vi "LSMcontroller_v60_PIzstage.vi"() -> ()   [LabVIEW 2015] (continued)
                                n921 = local write "img_CH2"(w3215) -> ()
                                n922 = local write "photons/frame"(w3208) -> ()
                                n923 = Array Max & Min(array=w3210) -> (max value=w3211:u16)  [unwired: 3 out]
                                n924 = To Single Precision Float(number=w3210) -> (single precision float=w3213:sgl[][])
                                n925 = case shown="True" w3222 {
                                tunnel: w3221 -> [_ w3226]
                                frame False {
                                }
                                frame True {
                                n926 = Quotient & Remainder(x=w3226, y=u32 2 ("min phot")) -> (floor(x/y)=w3225:u32)  [unwired: 1 out]
                                n927 = Max & Min(x=w3225, y=u32 5) -> (max(x,y)=w3224:u32)  [unwired: 1 out]
                                n928 = local write "min phot"(w3224) -> ()
                                }
                                }
                                n929 = To Double Precision Float(number=w3211) -> (double precision float=w3212:dbl)
                                n930 = local write "img_CH1"(w3213) -> ()
                                n931 = property on="img_CH1" class="IntGraph (strict)"("ZScale.Maximum"=w3212) -> ()  [unwired: 2 in, 2 out]
                                }
                                }
                                }
                                frame #4 {
                                w3230 = u16 1 items=["Stream to disk", "Post process", "real time process"] ("Ring")
                                n932 = local read "T3R Data processing"() -> (w3229:u16)
                                n933 = Equal?(x=w3229, y=w3230) -> (x = y?=w3228:bool)
                                n934 = case shown="False" w3228 {
                                frame False {
                                # "intensity"
                                n935 = local read "Current Average"() -> (w3235:sgl)
                                n936 = local read "image2list"() -> (w3231:u16)
                                n937 = local read "image1list"() -> (w3232:u16)
                                n938 = call "dattoimage.vi"("image2list"=w3231, "Current Average"=w3235, "image1list"=w3232) -> ("image 1 array out"=w3234:sgl[][])  [unwired: 1 out]
                                n939 = Transpose 2D Array(2D array=w3234) -> (transposed array=w3233:sgl[][])
                                n940 = local write "img_CH2"(w3233) -> ()
                                }
                                frame True {
                                }
                                }
                                }
                                }
                              }
                              frame Enabled {
                              }
                            }
                          }
                        }
                        n941 = local write "64bit disabled"(TRUE ("64bit disabled")) -> ()
                      }
                      frame #9 {
                        n942 = call "2pparameters.vi"("command"="get") -> ("params out"=w3238:T11)  [unwired: 1 in]
                        n943 = Unbundle By Name(w3238) -> ("auto OD"=w3237:bool)
                        n944 = case shown="True" w3237 {
                          frame False {
                          }
                          frame True {
                            n945 = call "configuration.vi"("command"="get") -> ("config out"=w3241:T12)  [unwired: 2 in, 1 out]
                            n946 = call "2pparameters.vi"("command"="get") -> ("params out"=w3244:T11)  [unwired: 1 in]
                            n947 = Unbundle By Name(w3241) -> ("image OD"=w3239:u16)
                            n948 = Unbundle By Name(w3244) -> ("ODfilt"=w3240:u16)
                            n949 = call "filterwheelcontrol_nothorlabslib.vi"("Current OD filt"=w3239, "New ODfilt"=w3240) -> ()  [unwired: 1 in]
                          }
                        }
                        n950 = call "reset AO_DO_v3.vi"() -> ()  [unwired: 12 in]
                      }
                      frame #10 {
                        n951 = stacked-sequence {
                          tunnel: w3258 -> [w3261 _ _ _ _ _]
                          tunnel: w3257 -> [w3260 _ _ _ _ _]
                          tunnel: w3256 -> [w3259 _ _ _ _ _]
                          tunnel: w3255 -> [_ w3310 _ _ _ _]
                          tunnel: w3254 -> [_ w3309 w3364 w3461 _ _]
                          tunnel: w3253 -> [_ w3308 w3363 w3460 _ _]
                          tunnel: w3252 -> [_ _ w3362 _ _ _]
                          tunnel: w3251 -> [_ _ w3361 _ _ _]
                          tunnel: w3250 -> [_ _ _ w3459 _ _]
                          tunnel: w3249 -> [_ _ _ w3458 _ _]
                          tunnel: w3248 -> [_ _ w3359 _ _ _]
                          tunnel: w3247 -> [_ _ w3358 _ _ _]
                          tunnel: w3246 -> [_ _ _ w3456 _ _]
                          tunnel: w3245 -> [_ _ _ w3455 _ _]
                          frame #0 {
                            n952 = case shown="False" w3261 {
                              tunnel: w3260 -> [_ w3283]
                              tunnel: w3259 -> [_ w3282]
                              frame True {
                                n953 = stacked-sequence {
                                seq-local: [w3262 _ _] -> [_ w3274 w3279]
                                frame #0 {
                                n954 = call "configuration.vi"("command"="get") -> ("config out"=w3268:T12)  [unwired: 2 in, 1 out]
                                n955 = Unbundle By Name(w3268) -> ("Voltage to Xgalvo"=w3265:i32)
                                n956 = call "2pparameters.vi"("command"="get") -> ("params out"=w3266:T11)  [unwired: 1 in]
                                n957 = in-place {
                                in-place-border: w3265 -> [w3273]
                                in-place-border: [w3270] -> w3262
                                n958 = in-place-cluster #9(w3266) -> ("aAO"=w3272:u32[])
                                n959 = call "remove channel from active arrayv2.vi"("line array in"=w3272, "line to remove"=w3273) -> ("line array out"=w3271:u32[], "index"=w3270:i32)  [unwired: 1 out]
                                n960 = in-place-cluster #9("aAO"=w3271) -> (w3263:T11)
                                }
                                n961 = call "2pparameters.vi"("Params in"=w3263, "command"="set") -> ()  [unwired: 1 out]
                                }
                                frame #1 {
                                n962 = call "waveformparamsv2.vi"("command"="rem AO", "index"=w3274) -> ()  [unwired: 3 in, 3 out]
                                }
                                frame #2 {
                                n963 = call "waveformsAObuffer.vi"("command"="get") -> ("AO wf out"=w3280:waveform(dbl)[])  [unwired: 1 in]
                                n964 = Delete From Array(array=w3280, length=1, index=w3279) -> (array with subset deleted=w3276:waveform(dbl)[])  [unwired: 1 out]
                                n965 = call "waveformsAObuffer.vi"("AO wf in"=w3276, "command"="set") -> ()  [unwired: 1 out]
                                }
                                }
                              }
                              frame False {
                                n966 = stacked-sequence {
                                seq-local: [w3284 _ _] -> [_ w3292 w3303]
                                tunnel: w3283 -> [_ w3291 _]
                                tunnel: w3282 -> [_ _ w3302]
                                frame #0 {
                                n967 = call "configuration.vi"("command"="get") -> ("config out"=w3289:T12)  [unwired: 2 in, 1 out]
                                n968 = Unbundle By Name(w3289) -> ("Voltage to Xgalvo"=w3285:i32)
                                n969 = call "2pparameters.vi"("command"="get") -> ("params out"=w3288:T11)  [unwired: 1 in]
                                n970 = Unbundle By Name(w3288) -> ("aAO"=w3286:u32[])
                                n971 = Search 1D Array(1D array=w3286, element=w3285) -> (index of element=w3284:i32)  [unwired: 1 in]
                                }
                                frame #1 {
                                n972 = call "waveformparamsv2.vi"("command"="get") -> ("Params out"=w3295:T15)  [unwired: 4 in, 2 out]
                                n973 = in-place {
                                in-place-border: w3292 -> [w3299]
                                in-place-border: w3291 -> [w3298]
                                n974 = in-place-cluster #10(w3295) -> ("AO parameters"=w3300:T16)
                                n975 = in-place {
                                in-place-border: w3298 -> [w3301]
                                n976 = in-place-array #11(w3300, w3299) -> ()  [unwired: 1 out]
                                n977 = in-place-array #11(w3301) -> (w3297:T16)  [unwired: 1 out]
                                }
                                n978 = in-place-cluster #10("AO parameters"=w3297) -> (w3293:T15)
                                }
                                n979 = call "waveformparamsv2.vi"("command"="set", "Params in"=w3293) -> ()  [unwired: 3 in, 3 out]
                                }
                                frame #2 {
                                n980 = call "waveformsAObuffer.vi"("command"="get") -> ("AO wf out"=w3306:waveform(dbl)[])  [unwired: 1 in]
                                n981 = Replace Array Subset(array=w3306, new element=w3302, index=w3303) -> (w3304:waveform(dbl)[])
                                n982 = call "waveformsAObuffer.vi"("AO wf in"=w3304, "command"="set") -> ()  [unwired: 1 out]
                                }
                                }
                              }
                            }
                          }
                          frame #1 {
                            n983 = case shown="True" w3310 {
                              tunnel: w3309 -> [_ w3332]
                              tunnel: w3308 -> [_ w3331]
                              frame True {
                                n984 = stacked-sequence {
                                seq-local: [w3311 _ _] -> [_ w3323 w3328]
                                frame #0 {
                                n985 = call "configuration.vi"("command"="get") -> ("config out"=w3317:T12)  [unwired: 2 in, 1 out]
                                n986 = Unbundle By Name(w3317) -> ("Voltage to Ygalvo"=w3314:i32)
                                n987 = call "2pparameters.vi"("command"="get") -> ("params out"=w3315:T11)  [unwired: 1 in]
                                n988 = in-place {
                                in-place-border: w3314 -> [w3322]
                                in-place-border: [w3319] -> w3311
                                n989 = in-place-cluster #12(w3315) -> ("aAO"=w3321:u32[])
                                n990 = call "remove channel from active arrayv2.vi"("line array in"=w3321, "line to remove"=w3322) -> ("line array out"=w3320:u32[], "index"=w3319:i32)  [unwired: 1 out]
                                n991 = in-place-cluster #12("aAO"=w3320) -> (w3312:T11)
                                }
                                n992 = call "2pparameters.vi"("Params in"=w3312, "command"="set") -> ()  [unwired: 1 out]
                                }
                                frame #1 {
                                n993 = call "waveformparamsv2.vi"("command"="rem AO", "index"=w3323) -> ()  [unwired: 3 in, 3 out]
                                }
                                frame #2 {
                                n994 = call "waveformsAObuffer.vi"("command"="get") -> ("AO wf out"=w3329:waveform(dbl)[])  [unwired: 1 in]
                                n995 = Delete From Array(array=w3329, length=1, index=w3328) -> (array with subset deleted=w3325:waveform(dbl)[])  [unwired: 1 out]
                                n996 = call "waveformsAObuffer.vi"("AO wf in"=w3325, "command"="set") -> ()  [unwired: 1 out]
                                }
                                }
                              }
                              frame False {
                                n997 = stacked-sequence {
                                seq-local: [w3333 _ _] -> [_ w3341 w3352]
                                tunnel: w3332 -> [_ w3340 _]
                                tunnel: w3331 -> [_ _ w3351]
                                frame #0 {
                                n998 = call "configuration.vi"("command"="get") -> ("config out"=w3338:T12)  [unwired: 2 in, 1 out]
                                n999 = Unbundle By Name(w3338) -> ("Voltage to Ygalvo"=w3334:i32)
                                n1000 = call "2pparameters.vi"("command"="get") -> ("params out"=w3337:T11)  [unwired: 1 in]
                                n1001 = Unbundle By Name(w3337) -> ("aAO"=w3335:u32[])
                                n1002 = Search 1D Array(1D array=w3335, element=w3334) -> (index of element=w3333:i32)  [unwired: 1 in]
                                }
                                frame #1 {
                                n1003 = call "waveformparamsv2.vi"("command"="get") -> ("Params out"=w3344:T15)  [unwired: 4 in, 2 out]
                                n1004 = in-place {
                                in-place-border: w3341 -> [w3348]
                                in-place-border: w3340 -> [w3347]
                                n1005 = in-place-cluster #13(w3344) -> ("AO parameters"=w3349:T16)
                                n1006 = in-place {
                                in-place-border: w3347 -> [w3350]
                                n1007 = in-place-array #14(w3349, w3348) -> ()  [unwired: 1 out]
                                n1008 = in-place-array #14(w3350) -> (w3346:T16)  [unwired: 1 out]
                                }
                                n1009 = in-place-cluster #13("AO parameters"=w3346) -> (w3342:T15)
                                }
                                n1010 = call "waveformparamsv2.vi"("command"="set", "Params in"=w3342) -> ()  [unwired: 3 in, 3 out]
                                }
                                frame #2 {
                                n1011 = call "waveformsAObuffer.vi"("command"="get") -> ("AO wf out"=w3355:waveform(dbl)[])  [unwired: 1 in]
                                n1012 = Replace Array Subset(array=w3355, new element=w3351, index=w3352) -> (w3353:waveform(dbl)[])
                                n1013 = call "waveformsAObuffer.vi"("AO wf in"=w3353, "command"="set") -> ()  [unwired: 1 out]
                                }
                                }
                              }
                            }
                          }
                          frame #2 {
                            n1014 = Build Array(w3359, w3358) -> (w3357:bool[])
                            n1015 = Boolean Array To Number(Boolean array=w3357) -> (number=w3360:u32)
                            n1016 = case shown="0" w3360 {
                              tunnel: w3364 -> [_ _ w3407]
                              tunnel: w3363 -> [_ _ w3406]
                              tunnel: w3362 -> [_ w3386 w3404]
                              tunnel: w3361 -> [_ w3385 w3405]
                              frame 1, Default {
                                n1017 = stacked-sequence {
                                seq-local: [w3365 _ _] -> [_ w3377 w3382]
                                frame #0 {
                                n1018 = call "configuration.vi"("command"="get") -> ("config out"=w3371:T12)  [unwired: 2 in, 1 out]
                                n1019 = Unbundle By Name(w3371) -> ("2P shutter"=w3368:i32)
                                n1020 = call "2pparameters.vi"("command"="get") -> ("params out"=w3369:T11)  [unwired: 1 in]
                                n1021 = in-place {
                                in-place-border: w3368 -> [w3376]
                                in-place-border: [w3373] -> w3365
                                n1022 = in-place-cluster #15(w3369) -> ("aDO"=w3375:u32[])
                                n1023 = call "remove channel from active arrayv2.vi"("line array in"=w3375, "line to remove"=w3376) -> ("line array out"=w3374:u32[], "index"=w3373:i32)  [unwired: 1 out]
                                n1024 = in-place-cluster #15("aDO"=w3374) -> (w3366:T11)
                                }
                                n1025 = call "2pparameters.vi"("Params in"=w3366, "command"="set") -> ()  [unwired: 1 out]
                                }
                                frame #1 {
                                n1026 = call "waveformparamsv2.vi"("command"="rem DO", "index"=w3377) -> ()  [unwired: 3 in, 3 out]
                                }
                                frame #2 {
                                n1027 = call "waveformsDObuffer.vi"("command"="get") -> ("DO wf out"=w3383:digitalwaveform[])  [unwired: 1 in]
                                n1028 = Delete From Array(array=w3383, length=1, index=w3382) -> (array with subset deleted=w3379:digitalwaveform[])  [unwired: 1 out]
                                n1029 = call "waveformsDObuffer.vi"("DO wf in"=w3379, "command"="set") -> ()  [unwired: 1 out]
                                }
                                }
                              }
                              frame 2 {
                                n1030 = stacked-sequence {
                                tunnel: w3386 -> [_ w3397 _]
                                tunnel: w3385 -> [_ _ w3401]
                                frame #0 {
                                n1031 = call "configuration.vi"("command"="get") -> ("config out"=w3388:T12)  [unwired: 2 in, 1 out]
                                n1032 = call "2pparameters.vi"("command"="get") -> ("params out"=w3392:T11)  [unwired: 1 in]
                                n1033 = Unbundle By Name(w3388) -> ("2P shutter"=w3387:i32)
                                n1034 = in-place {
                                in-place-border: w3387 -> [w3396]
                                n1035 = in-place-cluster #16(w3392) -> ("aDO"=w3395:u32[])
                                n1036 = call "add channel to active arrayv2.vi"("line array in"=w3395, "line to add"=w3396) -> ("line array out"=w3394:u32[])  [unwired: 2 out]
                                n1037 = in-place-cluster #16("aDO"=w3394) -> (w3390:T11)
                                }
                                n1038 = call "2pparameters.vi"("Params in"=w3390, "command"="set") -> ()  [unwired: 1 out]
                                }
                                frame #1 {
                                n1039 = call "waveformparamsv2.vi"("command"="add DO", "add DO"=w3397) -> ()  [unwired: 3 in, 3 out]
                                }
                                frame #2 {
                                n1040 = call "waveformsDObuffer.vi"("command"="get") -> ("DO wf out"=w3402:digitalwaveform[])  [unwired: 1 in]
                                n1041 = Build Array (concatenate)(w3402, w3401) -> (w3400:digitalwaveform[])
                                n1042 = call "waveformsDObuffer.vi"("DO wf in"=w3400, "command"="set") -> ()  [unwired: 1 out]
                                }
                                }
                              }
                              frame 0 {
                                n1043 = stacked-sequence {
                                seq-local: [w3408 _ _] -> [_ w3416 w3438]
                                tunnel: w3407 -> [_ _ _]
                                tunnel: w3406 -> [_ _ _]
                                tunnel: w3405 -> [_ _ w3437]
                                tunnel: w3404 -> [_ w3415 _]
                                frame #0 {
                                n1044 = call "configuration.vi"("command"="get") -> ("config out"=w3413:T12)  [unwired: 2 in, 1 out]
                                n1045 = call "2pparameters.vi"("command"="get") -> ("params out"=w3412:T11)  [unwired: 1 in]
                                n1046 = Unbundle By Name(w3413) -> ("2P shutter"=w3409:i32)
                                n1047 = Unbundle By Name(w3412) -> ("aDO"=w3410:u32[])
                                n1048 = Search 1D Array(1D array=w3410, element=w3409) -> (index of element=w3408:i32)  [unwired: 1 in]
                                }
                                frame #1 {
                                n1049 = call "2pparameters.vi"("command"="get") -> ("params out"=w3419:T11)  [unwired: 1 in]
                                n1050 = Unbundle By Name(w3419) -> ("wavdet"=w3417:bool, "autoshutter"=w3418:bool)
                                n1051 = case shown="True" w3418 {
                                tunnel: w3416 -> [_ w3423]
                                tunnel: w3417 -> [_ w3422]
                                tunnel: w3415 -> [_ w3421]
                                frame False {
                                }
                                frame True {
                                n1052 = case shown="False" w3422 {
                                tunnel: w3423 -> [w3427 _]
                                tunnel: w3421 -> [w3425 _]
                                frame False {
                                n1053 = Index Array(array=w3425, index=0) -> (element=w3424:T19)
                                n1054 = call "waveformparamsv2.vi"("command"="get") -> ("Params out"=w3430:T15)  [unwired: 4 in, 2 out]
                                n1055 = in-place {
                                in-place-border: w3427 -> [w3434]
                                in-place-border: w3424 -> [w3432]
                                n1056 = in-place-cluster #17(w3430) -> ("DO parameters"=w3435:T18)
                                n1057 = in-place {
                                in-place-border: w3432 -> [w3436]
                                n1058 = in-place-array #18(w3435, w3434) -> ()  [unwired: 1 out]
                                n1059 = in-place-array #18(w3436) -> (w3433:T18)  [unwired: 1 out]
                                }
                                n1060 = in-place-cluster #17("DO parameters"=w3433) -> (w3428:T15)
                                }
                                n1061 = call "waveformparamsv2.vi"("command"="set", "Params in"=w3428) -> ()  [unwired: 3 in, 3 out]
                                }
                                frame True {
                                }
                                }
                                }
                                }
                                }
                                frame #2 {
                                n1062 = call "2pparameters.vi"("command"="get") -> ("params out"=w3441:T11)  [unwired: 1 in]
                                n1063 = Unbundle By Name(w3441) -> ("wavdet"=w3439:bool, "autoshutter"=w3440:bool)
                                n1064 = case shown="True" w3440 {
                                tunnel: w3438 -> [_ w3445]
                                tunnel: w3439 -> [_ w3444]
                                tunnel: w3437 -> [_ w3443]
                                frame False {
                                }
                                frame True {
                                n1065 = case shown="False" w3444 {
                                tunnel: w3445 -> [w3449 _]
                                tunnel: w3443 -> [w3448 _]
                                frame False {
                                n1066 = Index Array(array=w3448, index=0) -> (element=w3446:digitalwaveform)
                                n1067 = call "waveformsDObuffer.vi"("command"="get") -> ("DO wf out"=w3451:digitalwaveform[])  [unwired: 1 in]
                                n1068 = Replace Array Subset(array=w3451, new element=w3446, index=w3449) -> (w3453:digitalwaveform[])
                                n1069 = call "waveformsDObuffer.vi"("DO wf in"=w3453, "command"="set") -> ()  [unwired: 1 out]
                                }
                                frame True {
                                }
                                }
                                }
                                }
                                }
                                }
                              }
                            }
                          }
                          frame #3 {
                            n1070 = Build Array(w3456, w3455) -> (w3457:bool[])
                            n1071 = Boolean Array To Number(Boolean array=w3457) -> (number=w3454:u32)
                            n1072 = case shown="0" w3454 {
                              tunnel: w3461 -> [_ _ w3504]
                              tunnel: w3460 -> [_ _ w3503]
                              tunnel: w3459 -> [_ w3483 w3501]
                              tunnel: w3458 -> [_ w3482 w3502]
                              frame 1, Default {
                                n1073 = stacked-sequence {
                                seq-local: [w3462 _ _] -> [_ w3474 w3479]
                                frame #0 {
                                n1074 = call "configuration.vi"("command"="get") -> ("config out"=w3468:T12)  [unwired: 2 in, 1 out]
                                n1075 = Unbundle By Name(w3468) -> ("LT timestamp"=w3465:u32)
                                n1076 = call "2pparameters.vi"("command"="get") -> ("params out"=w3466:T11)  [unwired: 1 in]
                                n1077 = in-place {
                                in-place-border: w3465 -> [w3473]
                                in-place-border: [w3470] -> w3462
                                n1078 = in-place-cluster #19(w3466) -> ("aDO"=w3472:u32[])
                                n1079 = call "remove channel from active arrayv2.vi"("line array in"=w3472, "line to remove"=w3473) -> ("line array out"=w3471:u32[], "index"=w3470:i32)  [unwired: 1 out]
                                n1080 = in-place-cluster #19("aDO"=w3471) -> (w3463:T11)
                                }
                                n1081 = call "2pparameters.vi"("Params in"=w3463, "command"="set") -> ()  [unwired: 1 out]
                                }
                                frame #1 {
                                n1082 = call "waveformparamsv2.vi"("command"="rem DO", "index"=w3474) -> ()  [unwired: 3 in, 3 out]
                                }
                                frame #2 {
                                n1083 = call "waveformsDObuffer.vi"("command"="get") -> ("DO wf out"=w3480:digitalwaveform[])  [unwired: 1 in]
                                n1084 = Delete From Array(array=w3480, length=1, index=w3479) -> (array with subset deleted=w3476:digitalwaveform[])  [unwired: 1 out]
                                n1085 = call "waveformsDObuffer.vi"("DO wf in"=w3476, "command"="set") -> ()  [unwired: 1 out]
                                }
                                }
                              }
                              frame 2 {
                                n1086 = stacked-sequence {
                                tunnel: w3483 -> [_ _ w3496]
                                tunnel: w3482 -> [_ w3494 _]
                                frame #0 {
                                n1087 = call "configuration.vi"("command"="get") -> ("config out"=w3485:T12)  [unwired: 2 in, 1 out]
                                n1088 = Unbundle By Name(w3485) -> ("LT timestamp"=w3484:u32)
                                n1089 = call "2pparameters.vi"("command"="get") -> ("params out"=w3489:T11)  [unwired: 1 in]
                                n1090 = in-place {
                                in-place-border: w3484 -> [w3493]
                                n1091 = in-place-cluster #20(w3489) -> ("aDO"=w3492:u32[])
                                n1092 = call "add channel to active arrayv2.vi"("line array in"=w3492, "line to add"=w3493) -> ("line array out"=w3491:u32[])  [unwired: 2 out]
                                n1093 = in-place-cluster #20("aDO"=w3491) -> (w3487:T11)
                                }
                                n1094 = call "2pparameters.vi"("Params in"=w3487, "command"="set") -> ()  [unwired: 1 out]
                                }
                                frame #1 {
                                n1095 = call "waveformparamsv2.vi"("command"="add DO", "add DO"=w3494) -> ()  [unwired: 3 in, 3 out]
                                }
                                frame #2 {
                                n1096 = call "waveformsDObuffer.vi"("command"="get") -> ("DO wf out"=w3499:digitalwaveform[])  [unwired: 1 in]
                                n1097 = Build Array (concatenate)(w3499, w3496) -> (w3498:digitalwaveform[])
                                n1098 = call "waveformsDObuffer.vi"("DO wf in"=w3498, "command"="set") -> ()  [unwired: 1 out]
                                }
                                }
                              }
                              frame 0 {
                                n1099 = stacked-sequence {
                                seq-local: [w3505 _ _] -> [_ w3515 w3532]
                                tunnel: w3504 -> [_ _ _]
                                tunnel: w3503 -> [_ _ _]
                                tunnel: w3502 -> [_ w3512 _]
                                tunnel: w3501 -> [_ _ w3531]
                                frame #0 {
                                n1100 = call "configuration.vi"("command"="get") -> ("config out"=w3510:T12)  [unwired: 2 in, 1 out]
                                n1101 = Unbundle By Name(w3510) -> ("LT timestamp"=w3506:u32)
                                n1102 = call "2pparameters.vi"("command"="get") -> ("params out"=w3509:T11)  [unwired: 1 in]
                                n1103 = Unbundle By Name(w3509) -> ("aDO"=w3507:u32[])
                                n1104 = Search 1D Array(1D array=w3507, element=w3506) -> (index of element=w3505:i32)  [unwired: 1 in]
                                }
                                frame #1 {
                                n1105 = local read "Measurement"() -> (w3514:T4)
                                n1106 = To Unsigned Long Integer(number=w3514) -> (unsigned 32bit integer=w3513:u32)
                                n1107 = case shown="5..7" w3513 {
                                tunnel: w3515 -> [_ w3519]
                                tunnel: w3512 -> [_ w3516]
                                frame 0..4, Default {
                                }
                                frame 5..7 {
                                n1108 = Index Array(array=w3516, index=0) -> (element=w3517:T19)
                                n1109 = call "waveformparamsv2.vi"("command"="get") -> ("Params out"=w3522:T15)  [unwired: 4 in, 2 out]
                                n1110 = in-place {
                                in-place-border: w3519 -> [w3526]
                                in-place-border: w3517 -> [w3524]
                                n1111 = in-place-cluster #21(w3522) -> ("DO parameters"=w3527:T18)
                                n1112 = in-place {
                                in-place-border: w3524 -> [w3528]
                                n1113 = in-place-array #22(w3527, w3526) -> ()  [unwired: 1 out]
                                n1114 = in-place-array #22(w3528) -> (w3525:T18)  [unwired: 1 out]
                                }
                                n1115 = in-place-cluster #21("DO parameters"=w3525) -> (w3520:T15)
                                }
                                n1116 = call "waveformparamsv2.vi"("command"="set", "Params in"=w3520) -> ()  [unwired: 3 in, 3 out]
                                }
                                }
                                }
                                frame #2 {
                                n1117 = local read "Measurement"() -> (w3530:T4)
                                n1118 = To Unsigned Long Integer(number=w3530) -> (unsigned 32bit integer=w3529:u32)
                                n1119 = case shown="5..7" w3529 {
                                tunnel: w3532 -> [_ w3536]
                                tunnel: w3531 -> [_ w3534]
                                frame 0..4, Default {
                                }
                                frame 5..7 {
                                n1120 = Index Array(array=w3534, index=0) -> (element=w3533:digitalwaveform)
                                n1121 = call "waveformsDObuffer.vi"("command"="get") -> ("DO wf out"=w3538:digitalwaveform[])  [unwired: 1 in]
                                n1122 = Replace Array Subset(array=w3538, new element=w3533, index=w3536) -> (w3540:digitalwaveform[])
                                n1123 = call "waveformsDObuffer.vi"("DO wf in"=w3540, "command"="set") -> ()  [unwired: 1 out]
                                }
                                }
                                }
                                }
                              }
                            }
                          }
                          frame #4 {
                            n1124 = call "Used AO lines.vi"() -> ("used AO names"=w3543:string[], "used AO lines"=w3541:tag[])  [unwired: 2 in]
                            n1125 = control-ref of="Analog Lines Plot"() -> (w3542:refnum<vi>)
                            n1126 = control-ref of="Digital Lines Plot"() -> (w3544:refnum<vi>)
                            n1127 = call "Used DO lines.vi"() -> ("used DO names"=w3545:string[], "used DO lines"=w3546:tag[])  [unwired: 2 in]
                            n1128 = local write "Analog Used Lines"(w3541) -> ()
                            n1129 = local write "Analog Used Names"(w3543) -> ()
                            n1130 = local write "Digital Used Lines"(w3546) -> ()
                            n1131 = local write "Digital Used Names"(w3545) -> ()
                            n1132 = call "prepDOWaveplot.vi"("DigitalGraph in"=w3544, "used DO names"=w3545) -> ()  [unwired: 1 in]
                            n1133 = call "prepAOWaveplot.vi"("WaveformGraph in"=w3542, "Analog Used Names"=w3543) -> ()  [unwired: 1 in]
                          }
                          frame #5 {
                            n1134 = local read "Meastab"() -> (w3561:enum32{"X-Y Image", "Linescan", "Timetrace"})
                            n1135 = property on="refwf" class="Ring (strict)"() -> ("RingText.Text"=w3558:string)  [unwired: 2 in, 2 out]
                            n1136 = case shown="\"Timetrace\"" w3561 {
                              tunnel: [w3563 w3564] -> w3562
                              frame "X-Y Image", Default {
                                n1137 = local read "Sampling rate"() -> (w3563:dbl)
                              }
                              frame "Timetrace" {
                                n1138 = local read "srateAODOtt"() -> (w3564:dbl)
                              }
                            }
                            n1139 = call "waveformsAObuffer.vi"("command"="get") -> ("AO wf out"=w3549:waveform(dbl)[])  [unwired: 1 in]
                            n1140 = local read "wavdet"() -> (w3559:bool)
                            n1141 = call "waveformsDObuffer.vi"("command"="get") -> ("DO wf out"=w3553:digitalwaveform[])  [unwired: 1 in]
                            n1142 = call "correctwaveformsizetemp.vi"("new sampling frequency (Hz)"=w3562, "start"=FALSE, "reference waveforms to"=w3558, "Analog waveforms in"=w3549, "stop"=TRUE, "Digital waveforms in"=w3553) -> ("analog wf out"=w3555:waveform(dbl)[], "Digital wf out"=w3557:digitalwaveform[], "measpoints"=w3560:i32)
                            n1143 = local write "Analog Lines Plot"(w3555) -> ()
                            n1144 = call "GetNumCamFramesv2.vi"("Digital Waveform Graph"=w3557) -> ("Numeric"=w3556:i32)  [unwired: 10 in]
                            n1145 = local write "Digital Lines Plot"(w3557) -> ()
                            n1146 = call "waveformsDObuffer.vi"("DO wf in"=w3557, "command"="set") -> ()  [unwired: 1 out]
                            n1147 = call "waveformsAObuffer.vi"("AO wf in"=w3555, "command"="set") -> ()  [unwired: 1 out]
                            n1148 = local write "Total Camera Frames"(w3556) -> ()
                            n1149 = case shown="True" w3559 {
                              tunnel: w3560 -> [_ w3565]
                              frame False {
                              }
                              frame True {
                                n1150 = local write "# of frames"(w3565) -> ()
                              }
                            }
                          }
                        }
                        n1151 = call "stoperaseCI.vi"() -> ()  [unwired: 12 in]
                        n1152 = call "stoperaseDO_img.vi"() -> ()  [unwired: 12 in]
                        n1153 = call "stoperaseAO_img.vi"() -> ()  [unwired: 12 in]
                        n1154 = call "stoperaseAI_img.vi"() -> ()  [unwired: 12 in]
                      }
                      frame #11 {
                        w3573 = FALSE ("Value (Signaling)")
                        n1155 = local read "save\ndata"() -> (w3566:bool)
                        n1156 = local read "save\ndata"() -> (w3567:bool)
                        n1157 = property on="Stop" class="Bool (strict)"("Visible"=FALSE, "DisabledEnum"=T7."Disabled" ("Disabled")) -> ()  [unwired: 2 in, 2 out]
                        n1158 = case shown="True" w3566 {
                          frame False {
                          }
                          frame True {
                            n1159 = call "closetiffs.vi"() -> ()  [unwired: 12 in]
                          }
                        }
                        n1160 = case shown="True" w3567 {
                          tunnel: w3568 -> [_ w3574]
                          frame False {
                          }
                          frame True {
                            n1161 = local read "filename prefix"() -> (w3576:string)
                            n1162 = local read "data dir"() -> (w3575:path)
                            n1163 = call "savetimestamps.vi"("timestamp"=w3574, "filename prefix in"=w3576, "data dir in"=w3575) -> ()  [unwired: 1 in]
                            n1164 = call "saveparams.vi"("filename prefix in"=w3576, "data dir in"=w3575) -> ()  [unwired: 2 in]
                          }
                        }
                        n1165 = property on="Start" class="Bool (strict)"("Visible"=TRUE, "DisabledEnum"=T7."Enabled" ("Disabled")) -> ()  [unwired: 2 in, 2 out]
                        n1166 = property on="Start" class="Bool (strict)"("Val(Sgnl)"=w3573) -> ()  [unwired: 2 in, 2 out]
                        n1167 = property on="Stop" class="Bool (strict)"("Val(Sgnl)"=w3573) -> ()  [unwired: 2 in, 2 out]
                      }
                      frame #12 {
                        w3580 = T22 2 items=["no dialog", "OK message", "continue or stop message", "OK message + warnings", "continue/stop + warnings"] ("type of dialog (OK msg:1)")
                        n1168 = call "displayerrors.vi"() -> ("error IO"=w3579:errorcluster)
                        n1169 = call <vilib>:"General Error Handler.vi"("type of dialog (OK msg:1)"=w3580, "error in (no error)"=w3579) -> ("error out"=w3578:errorcluster)  [unwired: 9 in, 4 out]
                        n1170 = call <vilib>:"Clear Errors.vi"("error in (no error)"=w3578) -> ("error out"=w3577:errorcluster)  [unwired: 5 in, 1 out]
                        n1171 = call "seterrors.vi"("error IO"=w3577) -> ()
                      }
                    }
                  }
                  frame "X-Y-Z-t movie" {
                    n1172 = call "2pparameters.vi"("command"="get") -> ("params out"=w3583:T11)  [unwired: 1 in]
                    n1173 = Bundle By Name(cluster=w3583, "type"="X-Y-Z-t movie") -> (w3581:T11)
                    n1174 = call "2pparameters.vi"("Params in"=w3581, "command"="set") -> ()  [unwired: 1 out]
                  }
                  frame "linescan" {
                    n1175 = call "2pparameters.vi"("command"="get") -> ("params out"=w3588:T11)  [unwired: 1 in]
                    n1176 = Bundle By Name(cluster=w3588, "type"="linescan") -> (w3590:T11)
                    n1177 = call "2pparameters.vi"("Params in"=w3590, "command"="set") -> ()  [unwired: 1 out]
                  }
                  frame "Timetrace", "Lifetime (contour)" {
                    n1178 = local read "ttt"() -> (w3591:T3)
                    n1179 = case shown="\"Resonant Ellipse\", \"freeform contour\"" w3591 {
                      frame "Point", Default {
                        n1180 = stacked-sequence {
                          seq-local: [w3592 _ _ _ _ _ _ _ _] -> [_ _ w3725 _ _ _ _ _ w3783]
                          frame #0 {
                            n1181 = Get Date/Time In Seconds() -> (seconds since 1Jan1904=w3593:timestamp)
                            n1182 = call "createdatafolder.vi"("timestamp in"=w3593) -> ("current data path"=w3594:path, "timestamp out"=w3592:timestamp)
                            n1183 = stacked-sequence {
                              frame #0 {
                                n1184 = call "2pparameters.vi"("command"="get") -> ("params out"=w3609:T11)  [unwired: 1 in]
                                n1185 = Bundle By Name(cluster=w3609, "type"="Timetrace") -> (w3607:T11)
                                n1186 = call "2pparameters.vi"("command"="get") -> ("params out"=w3598:T11)  [unwired: 1 in]
                                n1187 = local write "graphtab"(T5."timetrace" ("graphtab")) -> ()
                                n1188 = Unbundle By Name(w3598) -> ("Vx-min Img"=w3600:dbl, "VX-max Img"=w3599:dbl, "Vy-min Img"=w3602:dbl, "Vy-max Img"=w3601:dbl, "Angle Img"=w3603:dbl)
                                n1189 = property on="Stop" class="Bool (strict)"("Visible"=TRUE, "DisabledEnum"=T7."Enabled" ("Disabled")) -> ()  [unwired: 2 in, 2 out]
                                n1190 = property on="Start" class="Bool (strict)"("Visible"=FALSE, "DisabledEnum"=T7."Disabled and Grayed Out" ("Disabled")) -> ()  [unwired: 2 in, 2 out]
                                n1191 = local read "Vy-ref"() -> (w3605:dbl)
                                n1192 = local read "Vx-ref"() -> (w3604:dbl)
                                n1193 = call "2pparameters.vi"("Params in"=w3607, "command"="set") -> ()  [unwired: 1 out]
                                n1194 = script code="Xic=(ximax+ximin)./2;\nYic=(yimax+yimin)./2;\nx=x-Xic;\ny=y-Yic;\nxout=x.*cos(pi/180.*phi)+y.*sin(pi./180.*phi)+Xic;\nyout=-x.*sin(pi./180.*phi)+y.*cos(pi./180.*phi)+Yic;"("ximax"=w3599, "ximin"=w3600, "yimax"=w3601, "yimin"=w3602, "phi"=w3603, "x"=w3604, "y"=w3605) -> ("xout"=w3596:dbl, "yout"=w3595:dbl)  [unwired: 1 in, 1 out]
                                n1195 = call "setposition.vi"("Vy"=w3595, "Vx"=w3596) -> ()  [unwired: 1 in]
                              }
                              frame #1 {
                                n1196 = call "2pparameters.vi"("command"="get") -> ("params out"=w3618:T11)  [unwired: 1 in]
                                n1197 = Unbundle By Name(w3618) -> ("autoshutter"=w3619:bool, "auto OD"=w3616:bool)
                                n1198 = case shown="True" w3616 {
                                frame False {
                                }
                                frame True {
                                n1199 = call "configuration.vi"("command"="get") -> ("config out"=w3622:T12)  [unwired: 2 in, 1 out]
                                n1200 = Unbundle By Name(w3622) -> ("point OD"=w3623:u16)
                                n1201 = local read "ODfilt"() -> (w3620:u16)
                                n1202 = call "filterwheelcontrol_nothorlabslib.vi"("Current OD filt"=w3620, "New ODfilt"=w3623) -> ()  [unwired: 1 in]
                                }
                                }
                                n1203 = case shown="True" w3619 {
                                frame False {
                                }
                                frame True {
                                n1204 = call "shuttercontrol.vi"("command"="close") -> ()  [unwired: 1 in, 1 out]
                                }
                                }
                              }
                              frame #2 {
                                n1205 = local read "refreshtime"() -> (w3628:dbl)
                                n1206 = local read "wavdet"() -> (w3644:bool)
                                n1207 = local read "finite samples"() -> (w3643:bool)
                                n1208 = local read "srateAODOtt"() -> (w3629:dbl)
                                n1209 = local read "srateAODOtt"() -> (w3645:dbl)
                                n1210 = local read "srateAODOtt"() -> (w3630:dbl)
                                n1211 = Multiply(x=w3629, y=w3628) -> (x*y=w3639:dbl)
                                n1212 = local read "# of frames"() -> (w3638:i32)
                                n1213 = Reciprocal(x=w3628) -> (1/x=w3627:dbl)
                                n1214 = To Long Integer(number=w3639) -> (32bit integer=w3637:i32)
                                n1215 = Quotient & Remainder(x=w3638, y=w3637) -> (x-y*floor(x/y)=w3634:i32, floor(x/y)=w3631:i32)
                                n1216 = local read "AI channels"() -> (w3626:i32[])
                                n1217 = local read "CI channels"() -> (w3625:i32[])
                                n1218 = Equal To 0?(x=w3634) -> (x = 0?=w3633:bool)
                                n1219 = Increment(x=w3631) -> (x+1=w3632:i32)
                                n1220 = local read "continuous"() -> (w3642:bool)
                                n1221 = local read "Vx-ref"() -> (w3636:dbl)
                                n1222 = local read "Vy-ref"() -> (w3641:dbl)
                                n1223 = Select(t=w3631, s=w3633, f=w3632) -> (s? t:f=w3635:i32)
                                n1224 = local read "avpp"() -> (w3640:i32)
                                n1225 = call "2pparameters.vi"("command"="get") -> ("params out"=w3648:T11)  [unwired: 1 in]
                                n1226 = Bundle By Name(cluster=w3648, "measpoints"=w3638, "tt_cycles"=w3635, "refreshbuffer"=w3637, "refreshrate"=w3627, "Vx-ref"=w3636, "Vy-ref"=w3641, "srate"=w3645, "finite"=w3643, "cont"=w3642, "wavdet"=w3644, "avpp"=w3640, "srateAODO"=w3630, "aAI"=w3626, "aCI"=w3625) -> (w3646:T11)
                                n1227 = call "2pparameters.vi"("Params in"=w3646, "command"="set") -> ()  [unwired: 1 out]
                              }
                              frame #3 {
                                n1228 = local read "Vholding (mV)"() -> (w3651:sgl)
                                n1229 = local read "Current Clamp"() -> (w3657:bool)
                                n1230 = local read "Voltage Clamp"() -> (w3656:bool)
                                n1231 = local read "OCgain"() -> (w3652:sgl)
                                n1232 = local read "CC_ICgain"() -> (w3655:dbl)
                                n1233 = local read "holdon"() -> (w3650:bool)
                                n1234 = call "patchparameters.vi"("command"="get") -> ("Params out"=w3659:T14)  [unwired: 1 in]
                                n1235 = Bundle By Name(cluster=w3659, "VC"=w3656, "CC"=w3657, "CC_icg (pA/mv)"=w3655, "VC_icg (mV/mV)"=10.0, "OCG (mV/pA)"=w3652, "OVG (mV/mV)"=0.1, "Vhold (mV)"=w3651, "holdon"=w3650) -> (w3658:T14)
                                n1236 = call "patchparameters.vi"("Params in"=w3658, "command"="set") -> ()  [unwired: 1 out]
                              }
                              frame #4 {
                                n1237 = local read "wavdet"() -> (w3662:bool)
                                n1238 = case shown="True" w3662 {
                                frame False {
                                }
                                frame True {
                                n1239 = stacked-sequence {
                                frame #0 {
                                n1240 = disable-structure shown="Disabled" {
                                frame Disabled {
                                w3674 = 10178 items=["Finite Samples"=10178, "Continuous Samples"=10123, "Hardware Timed Single Point"=12522] ("sample mode")
                                n1241 = call "patchparameters.vi"("command"="get") -> ("Params out"=w3667:T14)  [unwired: 1 in]
                                n1242 = Unbundle By Name(w3667) -> ("CC"=w3668:bool)
                                n1243 = case shown="True" w3668 {
                                tunnel: [w3685 w3688] -> w3665
                                frame False {
                                n1244 = call "patchparameters.vi"("command"="get") -> ("Params out"=w3686:T14)  [unwired: 1 in]
                                n1245 = Unbundle By Name(w3686) -> ("VC_icg (mV/mV)"=w3685:sgl)
                                }
                                frame True {
                                n1246 = call "patchparameters.vi"("command"="get") -> ("Params out"=w3689:T14)  [unwired: 1 in]
                                n1247 = Unbundle By Name(w3689) -> ("CC_icg (pA/mv)"=w3688:sgl)
                                }
                                }
                                n1248 = local read "refreshtime"() -> (w3664:dbl)
                                n1249 = local read "srateAODOtt"() -> (w3675:dbl)
                                n1250 = local read item#-1() -> (w3678)
                                n1251 = local read item#-1() -> (w3684)
                                n1252 = local read item#-1() -> (w3677)
                                n1253 = local read item#-1() -> (w3682)
                                n1254 = local read item#-1() -> (w3676)
                                n1255 = local read item#-1() -> (w3683)
                                n1256 = local read item#-1() -> (w3681)
                                n1257 = local read item#-1() -> (w3679)
                                n1258 = local read item#-1() -> (w3680)
                                n1259 = Reciprocal(x=w3664) -> (1/x=w3663:dbl)
                                n1260 = call "waveformparamsv2.vi"("command"="get") -> ("Params out"=w3671:T23)  [unwired: 1 in]
                                n1261 = Bundle By Name(cluster=w3671, "AO parameters"=w3676, "DO parameters"=w3677, "Duty cycle sq(%)"=w3678, "Voltage freq. sq(Hz)"=w3679, "# cycles sq"=w3680, "meastype"=T9."Manual", "sample rate"=w3675, "amp"=w3665, "sample mode"=w3674, "Min Voltage tri (mV)"=w3681, "Max voltage tri (mV)"=w3682, "Voltage freq. tri(Hz)"=w3683, "# cycles tri"=w3684, "refreshrate"=w3663) -> (w3672:T23)
                                n1262 = call "waveformparamsv2.vi"("Params in"=w3672, "command"="set") -> ()  [unwired: 1 out]
                                }
                                frame Enabled {
                                }
                                }
                                }
                                frame #1 {
                                n1263 = disable-structure shown="Disabled" {
                                frame Disabled {
                                n1264 = call "2pparameters.vi"("command"="set") -> ("params out"=w3693:T11)  [unwired: 1 in]
                                n1265 = local read item#-1() -> (w3700)
                                n1266 = local read item#-1() -> (w3699)
                                n1267 = local read item#-1() -> (w3701)
                                n1268 = Unbundle By Name(w3693) -> ("aAO"=w3692:u32[], "aDO"=w3691:u32[])
                                n1269 = call "waveformparamsv2.vi"("command"="get") -> ("Params out"=w3697:T23)  [unwired: 1 in]
                                n1270 = Bundle By Name(cluster=w3697, "lAO"=w3692, "lDO"=w3691, "Voltage step"=w3699, "Voltage triangle"=w3701, "file"=w3700) -> (w3698:T23)
                                n1271 = call "waveformparamsv2.vi"("Params in"=w3698, "command"="set") -> ()  [unwired: 1 out]
                                }
                                frame Enabled {
                                }
                                }
                                }
                                frame #2 {
                                n1272 = disable-structure shown="Disabled" {
                                frame Disabled {
                                n1273 = local read item#-1() -> (w3703)
                                n1274 = call "load waveforms.vi"("waveform"=w3703) -> ("# of points"=w3702:i32)
                                n1275 = local write "# of frames"(w3702) -> ()
                                }
                                frame Enabled {
                                }
                                }
                                }
                                }
                                }
                                }
                              }
                              frame #5 {
                                n1276 = call "2pparameters.vi"("command"="get") -> ("params out"=w3714:T11)  [unwired: 1 in]
                                n1277 = Unbundle By Name(w3714) -> ("refreshbuffer"=w3712:i32, "srate"=w3713:sgl)
                                n1278 = local read "wavdet"() -> (w3706:bool)
                                n1279 = case shown="True" w3706 {
                                tunnel: [w3721 w3722] -> w3705
                                frame False {
                                w3721 = 10123 items=["Finite Samples"=10178, "Continuous Samples"=10123, "Hardware Timed Single Point"=12522] ("sample mode")
                                }
                                frame True {
                                w3722 = 10123 items=["Finite Samples"=10178, "Continuous Samples"=10123, "Hardware Timed Single Point"=12522] ("sample mode")
                                }
                                }
                                n1280 = To Double Precision Float(number=w3713) -> (double precision float=w3716:dbl)
                                n1281 = To Double Precision Float(number=w3712) -> (double precision float=w3707:dbl)
                                n1282 = Divide(x=w3707, y=w3716) -> (x/y=w3720:dbl)
                                n1283 = Multiply(x=w3720, y=2.0) -> (x*y=w3717:dbl)
                                n1284 = Max & Min(x=w3717, y=10.0) -> (max(x,y)=w3708:dbl)  [unwired: 1 out]
                                n1285 = call "2pparameters.vi"("command"="get") -> ("params out"=w3711:T11)  [unwired: 1 in]
                                n1286 = Bundle By Name(cluster=w3711, "timeout"=w3708, "sample mode"=w3705) -> (w3709:T11)
                                n1287 = call "2pparameters.vi"("Params in"=w3709, "command"="set") -> ()  [unwired: 1 out]
                              }
                            }
                            n1288 = local write "data dir"(w3594) -> ()
                          }
                          frame #1 {
                            # "determine size of AI buffer still!!!"
                            # "counter needs a clock. rather than setting up a separate clock line\n (i have no more counters) I opt to always record an AI channel;\nin imaging i don't do this because the scanner provides a clock and the\nspeed needed to record at appreciable framerates makes it useful to limit the number of channels.\nin timetrace, the samplerate is unlikely to ever go over >10Ks/s so it matters less."
                            # "shutter line"
                            # "to patch and\nlaser (eventual aotf)"
                            n1289 = call "prepAO_tt_v2.vi"() -> ("Terminal Name with Device Prefix"=w3723:tag)  [unwired: 2 in]
                            n1290 = call "prepDO_tt.vi"() -> ()  [unwired: 2 in]
                            n1291 = call "prepAI_ttv2.vi"("triggersource"=w3723) -> ()  [unwired: 1 in, 1 out]
                            n1292 = call "prepCI_tt.vi"() -> ()  [unwired: 2 in]
                          }
                          frame #2 {
                            n1293 = local read "save\ndata"() -> (w3724:bool)
                            n1294 = case shown="True" w3724 {
                              tunnel: w3725 -> [_ w3729]
                              frame False {
                              }
                              frame True {
                                n1295 = local read "filename prefix"() -> (w3727:string)
                                n1296 = local read "data dir"() -> (w3728:path)
                                n1297 = call "preparebinaryfiles.vi"("filename prefix"=w3727, "data dir"=w3728, "timestamp"=w3729) -> ("full-filename"=w3726:string)  [unwired: 1 in]
                                n1298 = local write "full-filename"(w3726) -> ()
                              }
                            }
                          }
                          frame #3 {
                            n1299 = call "2pparameters.vi"("command"="get") -> ("params out"=w3731:T11)  [unwired: 1 in]
                            n1300 = Unbundle By Name(w3731) -> ("autoshutter"=w3732:bool)
                            n1301 = case shown="True" w3732 {
                              frame False {
                              }
                              frame True {
                                n1302 = call "shuttercontrol.vi"("command"="open") -> ()  [unwired: 1 in, 1 out]
                              }
                            }
                          }
                          frame #4 {
                            n1303 = flat-sequence {
                              frame #0 {
                                n1304 = call "runAI_img.vi"() -> ()  [unwired: 12 in]
                                n1305 = call "runCI.vi"() -> ()  [unwired: 12 in]
                                n1306 = call "runDO_img.vi"() -> ()  [unwired: 12 in]
                                n1307 = call "runAO_img.vi"() -> ()  [unwired: 12 in]
                              }
                              frame #1 {
                              }
                            }
                          }
                          frame #5 {
                            n1308 = while {
                              i -> [w3736]
                              stop <- w3734 stop-if-true
                              n1309 = local read "Stop"() -> (w3744:bool)
                              n1310 = local read "Exit"() -> (w3743:bool)
                              n1311 = Increment(x=w3736) -> (x+1=w3735:i32)
                              n1312 = local write "points recorded"(w3735) -> ()
                              n1313 = Or(x=w3744, y=w3743) -> (x .or. y?=w3742:bool)
                              n1314 = case shown="False" w3742 {
                                frame False {
                                n1315 = stacked-sequence {
                                frame #0 {
                                n1316 = call "collectCI_tt.vi"() -> ("size(s)"=w3751:i32)  [unwired: 3 in]
                                n1317 = local write "scol"(w3751) -> ()
                                n1318 = call "collectAI_tt_V2.vi"() -> ()  [unwired: 4 in]
                                }
                                frame #1 {
                                n1319 = local read "graph2list"() -> (w3756:u16)
                                n1320 = local read "graph1list"() -> (w3757:u16)
                                n1321 = To Unsigned Word Integer(number=w3756) -> (unsigned 16bit integer=w3759:u16)
                                n1322 = To Unsigned Word Integer(number=w3757) -> (unsigned 16bit integer=w3760:u16)
                                n1323 = local read "bin"() -> (w3764:dbl)
                                n1324 = call "dattotrace.vi"("graph2list"=w3759, "Current Average"=sgl 1.0, "graph1list"=w3760) -> ("trace2array out"=w3762:sgl[], "trace1array out"=w3761:sgl[])
                                n1325 = Array Size(array=w3762) -> (size(s)=w3765:i32)
                                n1326 = Divide(x=w3765, y=2) -> (x/y=w3767:dbl)
                                n1327 = Round To Nearest(number=w3767) -> (nearest integer value=w3769:dbl)
                                n1328 = script code="data=reshape(datain,[bin length(datain)./bin]);\ndataout=mean(data,1);"("bin"=w3764, "datain"=w3761) -> ("dataout"=w3763:dbl[])  [unwired: 1 in, 1 out]
                                n1329 = Array Size(array=w3763) -> (size(s)=w3774:i32)
                                n1330 = Delete From Array(array=w3762, length=w3769, index=0) -> (deleted portion=w3753:sgl[], array with subset deleted=w3752:sgl[])
                                n1331 = Divide(x=w3774, y=2) -> (x/y=w3772:dbl)
                                n1332 = Round To Nearest(number=w3772) -> (nearest integer value=w3770:dbl)
                                n1333 = Delete From Array(array=w3763, length=w3770, index=0) -> (deleted portion=w3754:dbl[], array with subset deleted=w3755:dbl[])
                                n1334 = local write "graph4"(w3752) -> ()
                                n1335 = local write "graph2"(w3755) -> ()
                                n1336 = local write "graph3"(w3753) -> ()
                                n1337 = local write "graph1"(w3754) -> ()
                                }
                                frame #2 {
                                n1338 = local read "save\ndata"() -> (w3775:bool)
                                n1339 = case shown="True" w3775 {
                                frame False {
                                }
                                frame True {
                                n1340 = call "savebinaryfiles.vi"() -> ()  [unwired: 1 in]
                                }
                                }
                                }
                                }
                                }
                                frame True {
                                }
                              }
                              n1341 = local read "continuous"() -> (w3739:bool)
                              n1342 = case shown="False" w3739 {
                                tunnel: w3735 -> [w3749 _]
                                tunnel: [w3748 FALSE] -> w3737
                                frame False {
                                n1343 = call "2pparameters.vi"("command"="get") -> ("params out"=w3746:T11)  [unwired: 1 in]
                                n1344 = Unbundle By Name(w3746) -> ("tt_cycles"=w3745:i32)
                                n1345 = Greater Or Equal?(x=w3749, y=w3745) -> (x >= y?=w3748:bool)
                                }
                                frame True {
                                }
                              }
                              n1346 = local read "Stop"() -> (w3741:bool)
                              n1347 = local read "Exit"() -> (w3740:bool)
                              n1348 = Or(x=w3741, y=w3740) -> (x .or. y?=w3738:bool)
                              n1349 = Or(x=w3738, y=w3737) -> (x .or. y?=w3734:bool)
                            }
                          }
                          frame #6 {
                            n1350 = call "stoperaseCI.vi"() -> ()  [unwired: 12 in]
